vi "lvparse perf test.vi"() -> ()   [LabVIEW 2014]
uses:
  test2json.ctl
panel:
  out "x-y":dbl
  out "value":T1
  in  "String":string="{\n    \"id\": 1,\n    \"name\": \"Foo\",\n    \"price\": 123,\n    \"tags\": [ \"Bar\", \"Eek\" ],\n    \"stock\": {\n        \"warehouse\": 300,\n        \"retail\": 20\n    }\n}"
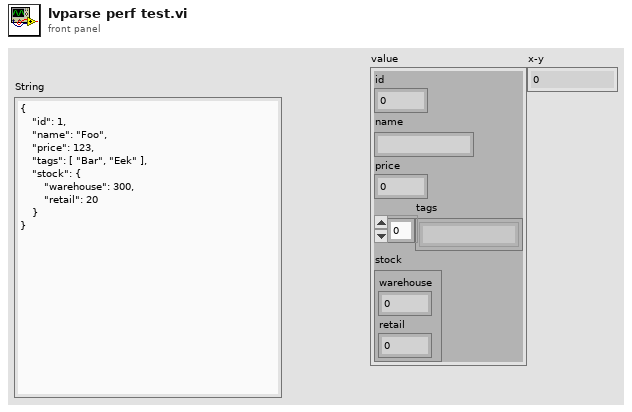
[diagram p1: front panel]
types:
  T1 = typedef "test2json.ctl" = cluster{"id":i32, "name":string, "price":i32, "tags":string[], "stock":cluster{"warehouse":i32, "retail":i32}}
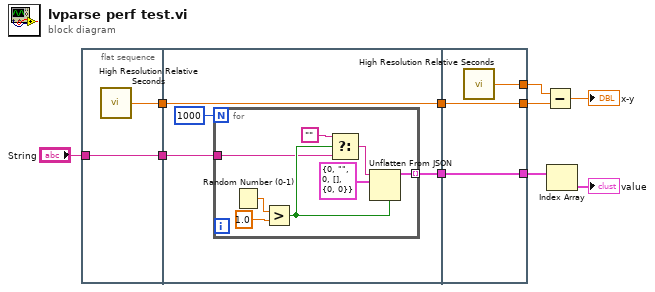
[diagram p0: block diagram]
diagram:
  n1 = flat-sequence {
    tunnel: "String" -> [w12]
    tunnel: [w12] -> w7
    tunnel: [w11] -> w5
    tunnel: [w15] -> w8
    tunnel: w7 -> [w16]
    tunnel: w5 -> [w14]
    tunnel: [w14] -> w4
    tunnel: [w27] -> w9
    tunnel: w8 -> [w27]
    tunnel: [w26] -> w6
    tunnel: w4 -> [w25]
    tunnel: [w25] -> w3
    frame #0 {
      n2 = call <vilib>:"High Resolution Relative Seconds.vi"() -> ("relative seconds"=w11:dbl)
    }
    frame #1 {
      n3 = for {
        N: 1000 -> [_]
        tunnel: w16 -> [w18]
        tunnel: [w23] -> w15 mode=indexing
        n4 = Random Number (0-1)() -> (number: 0 to 1=w22:dbl)
        n5 = Greater?(x=w22, y=1.0) -> (0:w20:bool)
        n6 = Select(t="", s=w20, f=w18) -> (s? t:f=w17:string)
        n7 = Unflatten From JSON(JSON string=w17, type and defaults=T1 {"id"=0, "name"="", "price"=0, "tags"=[], "stock"={"warehouse"=0, "retail"=0}}, strict validation? (F)=w20) -> (value=w23:T1)  [unwired: 4 in, 1 out]
      }
    }
    frame #2 {
      n8 = call <vilib>:"High Resolution Relative Seconds.vi"() -> ("relative seconds"=w26:dbl)
    }
  }
  n9 = Subtract(x=w6, y=w3) -> (x-y=→"x-y":dbl)
  n10 = Index Array(array=w9) -> (element=→"value":T1)  [unwired: 1 in]
